vi "Actor Core.vi"(8 "error in":errorcluster, 11 "Instrument in":refnum<class "Instrument.lvclass">) -> (0 "error out":errorcluster, 3 "Actor out":refnum<class "Actor.lvclass">)   [LabVIEW 2020, in "2. Basic Panel Actors.lvlib" / "Instrument.lvclass"]
doc: "The user interface for this panel.\n----\nCopyright: MGI 2016\nAuthor: Derek Trepanier"
uses:
  Instrument.lvclass
  C:/Program Files/National Instruments/LabVIEW 2020/vi.lib/MGI/Panel Manager/Panel Actor/Panel Actor/Panel Actor.lvclass
  <vilib>/ActorFramework/Actor/Actor.lvclass
  <vilib>/MGI/Panel Manager/Panel/Panel Helper/Panel Helper.lvclass/Panel Helper.ctl
  <vilib>/ActorFramework/Message Enqueuer/Message Enqueuer.lvclass/Message Enqueuer.ctl
  <vilib>/ActorFramework/Message Enqueuer/Enqueue.vi
  <vilib>/MGI/Panel Manager/Panel/Panel/Subpanel/Subpanel.lvclass
  C:/Program Files/National Instruments/LabVIEW 2020/vi.lib/MGI/Panel Manager/Panel/Panel/Panel.lvclass
  <vilib>/ActorFramework/Stop Msg/Stop Msg.lvclass
  C:/Program Files/National Instruments/LabVIEW 2020/vi.lib/ActorFramework/Message/Message.lvclass
  <vilib>/MGI/Panel Manager/Panel/Panel/Subpanel/Subpanel.vi
  <vilib>/ActorFramework/Message Priority Queue/Priority Enqueue.vi
  <vilib>/MGI/Panel Manager/Panel/Panel Updater/Panel Updater.lvclass
  <vilib>/MGI/Panel Manager/Panel Actor/Panel Actor/Panel Actor.lvclass
  <vilib>/MGI/Panel Manager/Panel/Panel.lvlib
  <vilib>/MGI/Panel Manager/Panel/Panel Helper/Panel Helper.lvclass
panel:
  in  "Name":string
  out "ID":string
  in  "Save":bool
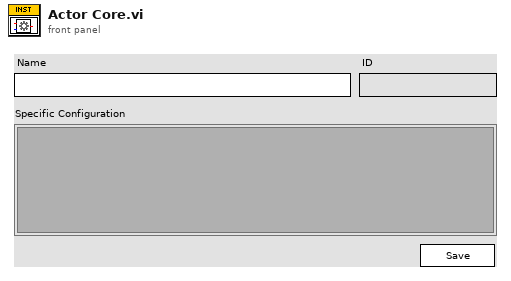
[diagram p1: front panel]
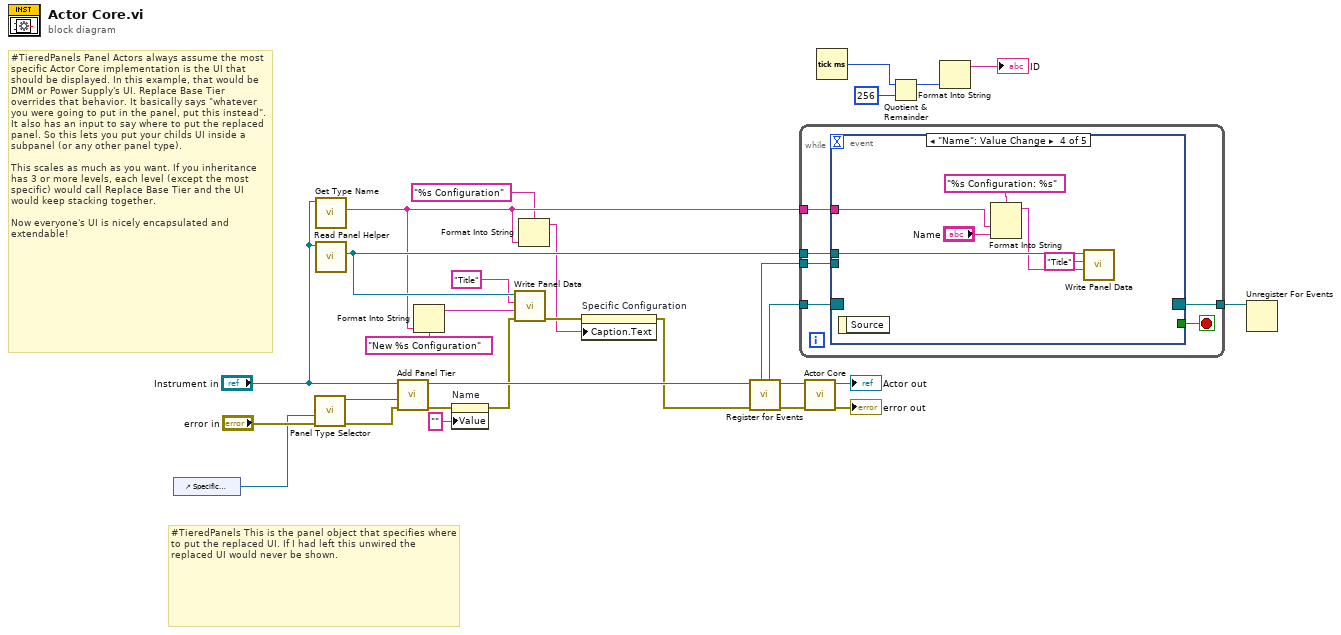
[diagram p0: block diagram]
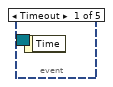
[diagram p2: hidden frame]
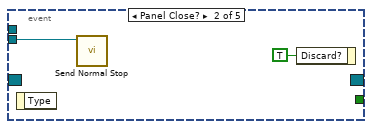
[diagram p3: hidden frame]
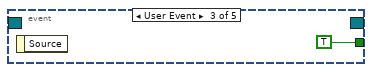
[diagram p4: hidden frame]
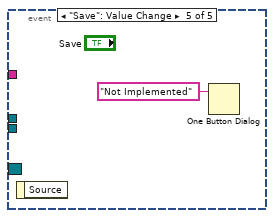
[diagram p5: hidden frame]
diagram:
  # "#TieredPanels This is the panel object that specifies where to put the replaced UI. If I had left this unwired the replaced UI would never be shown."
  # "#TieredPanels Panel Actors always assume the most specific Actor Core implementation is the UI that should be displayed. In this example, that would be DMM or Power Supply's UI. Replace Base Tier overrides that behavior. It basically says \"whatever you were going to put in the panel, put this instead\". It also has an input to say where to put the replaced panel. So this lets you put your childs UI inside a subpanel (or any other panel type).\n\nThis scales as much as you want. If you inheritance has 3 or more levels, each level (except the most specific) would call Replace Base Tier and the UI would keep stacking together.\n\nNow everyone's UI is nicely encapsulated and extendable!"
  n1 = control-ref of="Specific Configuration"() -> (w24:refnum<vi>)
  n2 = call-poly <vilib>:"Panel Type Selector.vi"("Error In"="error in", "Sub Panel"=w24) -> ("Error Out"=w25:errorcluster, "Subpanel Out"=w27:refnum<class "Subpanel.lvclass">)  [unwired: 8 in]
  n3 = call-dynamic "Get Type Name.vi"("Instrument in"="Instrument in") -> ("Type Name"=w4:string)  [unwired: 10 in]
  n4 = call <vilib>:"Read Panel Helper.vi"("Panel Actor in"="Instrument in") -> ("Panel Helper"=w11:refnum<class "Panel Helper.lvclass">)  [unwired: 9 in, 1 out]
  n5 = call <vilib>:"Add Panel Tier.vi"("Error In"=w25, "Old VI's Destination"=w27, "Panel Actor in"="Instrument in") -> ("Error Out"=w14:errorcluster, "Panel Actor out"=w22:refnum<class "Instrument.lvclass">)  [unwired: 7 in]
  n6 = Format Into String(format string="New %s Configuration", w4) -> (resulting string=w7:string)  [unwired: 2 in, 1 out]
  n7 = property on="Name" class="Str"(error in=w14, "Value"="" ("Name")) -> (error out=w10:errorcluster)  [unwired: 1 in, 1 out]
  n8 = call <vilib>:"Write Panel Data.vi"("Error In"=w10, "Panel Data"=w7, "Field"="Title", "Panel Helper in"=w11) -> ("Error Out"=w6:errorcluster)  [unwired: 6 in, 1 out]
  n9 = Format Into String(format string="%s Configuration", w4) -> (resulting string=w2:string)  [unwired: 2 in, 1 out]
  n10 = property on="Specific Configuration" class="SubPnl"(error in=w6, "Caption.Text"=w2) -> (error out=w5:errorcluster)  [unwired: 1 in, 1 out]
  n11 = call <vilib>:"Register for Events.vi"("Error In"=w5, "Panel Actor in"=w22) -> ("Error Out"=w23:errorcluster, "Panel Actor out"=w21:refnum<class "Instrument.lvclass">, "Pnl Actor"=w20:refnum<event-registration>, "Self Enqueuer"=w19:refnum<class "Message Enqueuer.lvclass">)  [unwired: 6 in]
  n12 = while {
    tunnel: w20 -> [w35]
    tunnel: w19 -> [w34]
    tunnel: w4 -> [w32]
    tunnel: w11 -> [w31]
    tunnel: [w30] -> w1
    stop <- w33 stop-if-true
    n13 = event shown="[3] \"Name\": Value Change" {
      selector: w35 -> [_ _ _ _ _]
      dyn-events: [_ _ _ _ _] -> w30
      timeout: _ -> [_ _ _ _ _]
      tunnel: w34 -> [_ w37 _ _ _]
      tunnel: [_ _ TRUE _ _] -> w33
      tunnel: w32 -> [_ _ _ w43 _]
      tunnel: w31 -> [_ _ _ w42 _]
      event Timeout {
        n14 = event-data() -> ()  [unwired: 1 in, 1 out]
      }
      event Panel Close? {
        n15 = event-data() -> ()  [unwired: 1 in, 1 out]
        n16 = call <vilib>:"Send Normal Stop.vi"("Message Enqueuer"=w37) -> ()  [unwired: 10 in, 1 out]
        n17 = event-data("Discard?"=TRUE) -> ()  [unwired: 1 in, 1 out]
      }
      event User Event {
        n18 = event-data() -> ()  [unwired: 1 in, 1 out]
      }
      event "Name": Value Change {
        n19 = event-data() -> ()  [unwired: 1 in, 1 out]
        n20 = Format Into String(format string="%s Configuration: %s", w43, "Name") -> (resulting string=w41:string)  [unwired: 2 in, 1 out]
        n21 = call <vilib>:"Write Panel Data.vi"("Panel Data"=w41, "Field"="Title", "Panel Helper in"=w42) -> ()  [unwired: 7 in, 2 out]
      }
      event "Save": Value Change {
        n22 = event-data() -> ()  [unwired: 1 in, 1 out]
        n23 = One Button Dialog(message="Not Implemented") -> ()  [unwired: 1 in, 1 out]
      }
    }
  }
  n24 = call-parent "Actor Core.vi"("error in"=w23, "Panel Actor in"=w21) -> ("error out"=→"error out":errorcluster, "Actor out"=→"Actor out":refnum<class "Actor.lvclass">)  [unwired: 8 in]
  n25 = Tick Count (ms)() -> (millisecond timer value=w18:u32)
  n26 = Quotient & Remainder(x=w18, y=u32 256) -> (x-y*floor(x/y)=w16:u32)  [unwired: 1 out]
  n27 = Format Into String(w16) -> (resulting string=→"ID":string)  [unwired: 3 in, 1 out]
  n28 = Unregister For Events(event registration refnum=w1) -> ()  [unwired: 1 in, 1 out]
